vi "v2 get num dockingstations on host.vi"(11 "num_devices":u32) -> (2 "function return":i32, 3 "num_devices out":u32)   [LabVIEW 2019, in "apdm.lvlib"]
doc: "APDM_EXPORT int apdm_v2_get_num_dockingstations_on_host(uint32_t *num_devices);"
uses:
  apdm.lvlib
  Lee Lab/CP FES Walking 2018/Code/Working/LabVIEW/apdm.dll
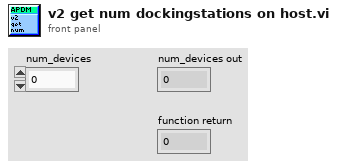
[diagram p1: front panel]
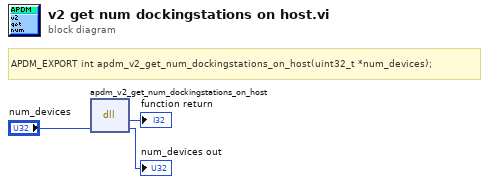
[diagram p0: block diagram]
diagram:
  # "APDM_EXPORT int apdm_v2_get_num_dockingstations_on_host(uint32_t *num_devices);"
  n1 = dll-call lib="C:/Users/jfalesi/Dropbox/Lee Lab/CP FES Walking 2018/Code/Working/LabVIEW/apdm.*" fn="apdm_v2_get_num_dockingstations_on_host"("num_devices"="num_devices") -> (→"function return":i32, "num_devices"=→"num_devices out":u32)  [unwired: 3 in, 2 out]
